vi "fit -- freq vs T - V3.vi"(0 "time points":dbl[](array[numeric]), 1 "varshni win (relative)":dbl=1.25, 2 "fit using":T1=enum."varshni", 5 "temperature points":dbl[](array[numeric]), 9 "frequency points":dbl[](array[numeric]), 11 "cursor bracket: freq":T2={"left"=2378.60310421286, "right "=2421.6740576496672, "center"=2421.6740576496672, "window"=2421.6740576496672, "cursors"=[], "relative"=0, "absolute"=0, "fixed vertical offset"=2421.6740576496672, "vertical offset"=2421.6740576496672, "skew"=2421.6740576496672, "default window frac"=2421.6740576496672, "kind"=enum."skewed", "skew.left"=2421.6740576496672, "skew.right"=2421.6740576496672, "Plot ref"=refnum, "wing order"=enum."back"}, 12 "redo for varshni window?":bool) -> (3 "best fit parameters":dbl[](array[numeric])=[1510.033618014085, -0.06734487332989668, -59.94387240978006], 4 "fit function name":string="fit function - varshni3.vi", 13 "fit points before":i32=434, 14 "fit points after":i32=434)   [LabVIEW 2015]
uses:
  D:/github/resonant_ultrasound/maglab ultrasound -- arkady/cursor winow.ctl
  fit function selector control.ctl
  <vilib>/gmath/NumericalOptimization/Nonlinear Curve Fit LM.vi
  <vilib>/gmath/NI_Gmath.lvlib
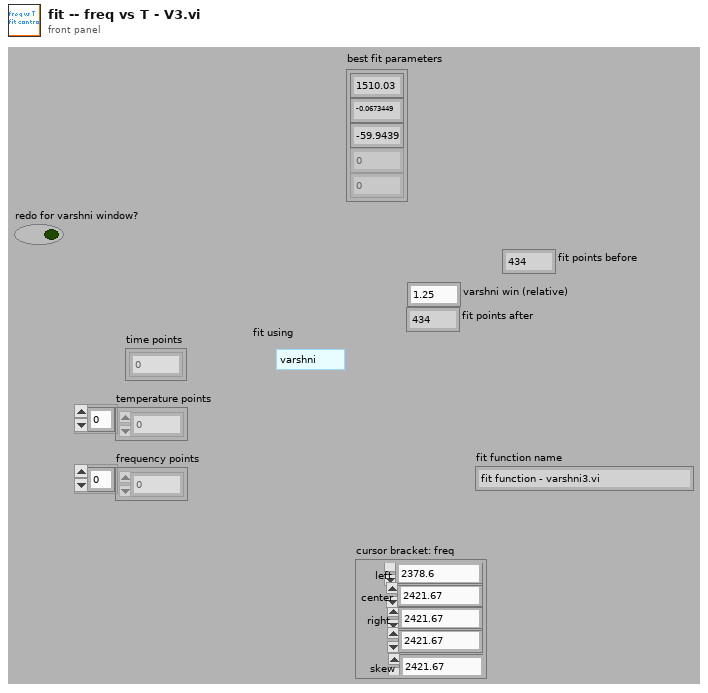
[diagram p1: front panel]
types:
  T1 = typedef "fit function selector control.ctl" = enum16{"linear", "varshni", "varshni5", "LogMinusT", "hyperbola", "einstein", "sine", "sine2theta", "cos2theta"}
  T2 = typedef "cursor winow.ctl" = cluster{"left":dbl, "right ":dbl, "center":dbl, "window":dbl, "cursors":i32[], "relative":i32, "absolute":i32, "fixed vertical offset":dbl, "vertical offset":dbl, "skew":dbl, "default window frac":dbl, "kind":enum16{"symmetric", "skewed", "fancy"}, "skew.left":dbl, "skew.right":dbl, "Plot ref":refnum<vi>, "wing order":enum16{"forw", "back"}}
  T3 = cluster{"model":string, "Parameters":string[], "x":string}
  T4 = typedef "NI_Gmath.lvlib/LM model function reference.ctl" = refnum<vi>
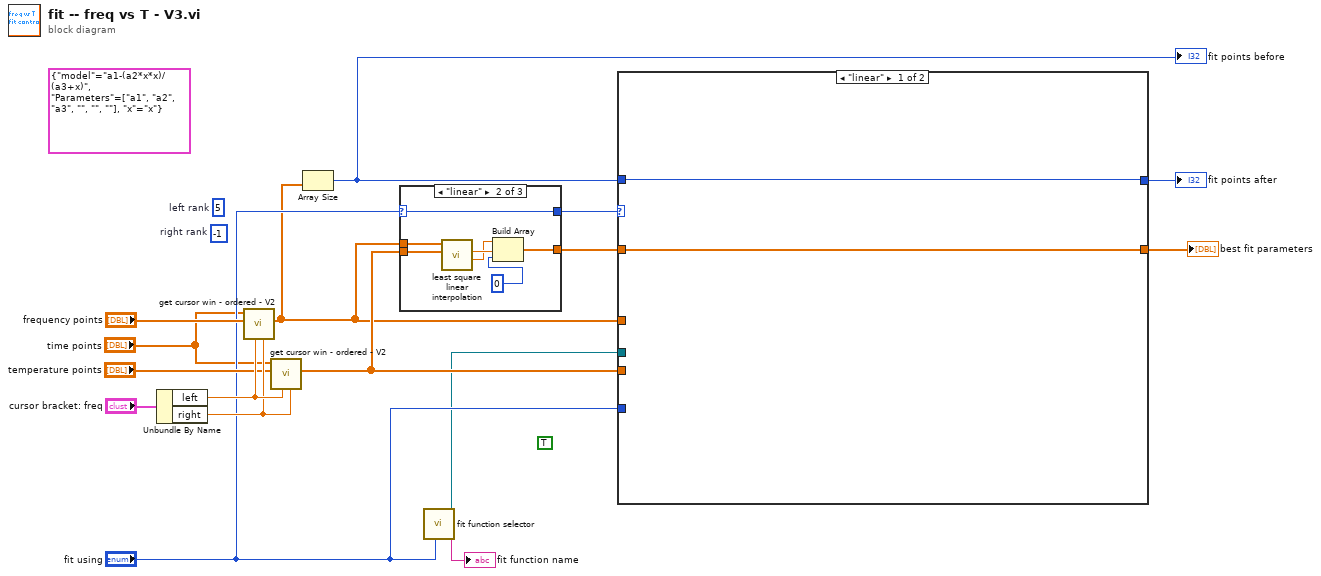
[diagram p0: block diagram]
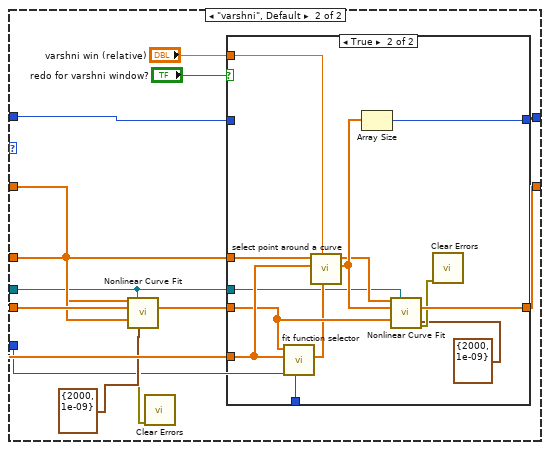
[diagram p2: hidden frame]
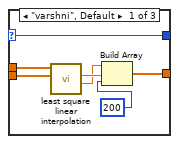
[diagram p4: hidden frame]
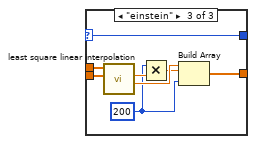
[diagram p5: hidden frame]
diagram:
  (unwired) T3 {"model"="a1-(a2*x*x)/(a3+x)", "Parameters"=["a1", "a2", "a3", "", "", ""], "x"="x"} ("model description")
  (unwired) TRUE
  (unwired) -1  # right rank
  (unwired) 5  # left rank
  n1 = Unbundle By Name("cursor bracket: freq") -> ("left"=w14:dbl, "right"=w13:dbl)
  n2 = call "get cursor win - ordered - V2.vi"("right"=w13, "left"=w14, "freq"="frequency points", "time points"="time points") -> ("freq out"=w4:dbl[])  [unwired: 6 in, 1 out]
  n3 = call "get cursor win - ordered - V2.vi"("right"=w13, "left"=w14, "freq"="temperature points", "time points"="time points") -> ("freq out"=w9:dbl[])  [unwired: 6 in, 1 out]
  n4 = Array Size(array=w4) -> (size(s)=w2:i32)
  "fit points before" <- w2
  n5 = case shown="\"linear\"" "fit using" {
    selector: "fit using" -> [w17 w24 w31]
    tunnel: w9 -> [w23 w30 w38]
    tunnel: w4 -> [w22 w29 w37]
    tunnel: [w20 w27 w36] -> w8
    tunnel: [w17 w24 w31] -> w1
    frame "varshni", Default {
      n6 = call "least square linear interpolation.vi"("X"=w23, "Y"=w22) -> ("intercept"=w18:dbl, "slope"=w19:dbl)  [unwired: 8 in]
      n7 = Build Array(w18, w19, 200) -> (w20:dbl[])
    }
    frame "linear" {
      n8 = call "least square linear interpolation.vi"("X"=w30, "Y"=w29) -> ("intercept"=w25:dbl, "slope"=w26:dbl)  [unwired: 8 in]
      n9 = Build Array(w25, w26, 0) -> (w27:dbl[])
    }
    frame "einstein" {
      w33 = 200
      n10 = call "least square linear interpolation.vi"("X"=w38, "Y"=w37) -> ("intercept"=w35:dbl, "slope"=w34:dbl)  [unwired: 8 in]
      n11 = Multiply(x=w33, y=w34) -> (x*y=w32:dbl)
      n12 = Build Array(w35, w32, w33) -> (w36:dbl[])
    }
  }
  n13 = call "fit function selector.vi"("fit using"="fit using") -> ("fit function name"=→"fit function name":string, "vi reference"=w3:T4)  [unwired: 8 in, 1 out]
  n14 = case shown="\"linear\"" w1 {
    tunnel: [w40 w52] -> w12
    tunnel: [w39 w51] -> w11
    tunnel: w9 -> [_ w50]
    tunnel: w8 -> [w40 w46]
    tunnel: "fit using" -> [_ w45]
    tunnel: w4 -> [_ w44]
    tunnel: w3 -> [_ w43]
    tunnel: w2 -> [w39 w41]
    frame "linear" {
    }
    frame "varshni", Default {
      n15 = call-poly <vilib>:"Nonlinear Curve Fit.vi"("Y"=w44, "f(x,a)"=w43, "X"=w50, "initial parameters"=w46, "termination"=cluster{"max iteration":i32, "tolerance":dbl} {"max iteration"=2000, "tolerance"=1e-09}) -> ("best fit parameters"=w47:dbl[], "error out"=w48:errorcluster)  [unwired: 5 in, 4 out]
      n16 = call <vilib>:"Clear Errors.vi"("error in (no error)"=w48) -> ()  [unwired: 5 in, 2 out]
      n17 = case shown="True" "redo for varshni window?" {
        tunnel: "varshni win (relative)" -> [_ w68]
        tunnel: [w55 w67] -> w52
        tunnel: [w54 w66] -> w51
        tunnel: w50 -> [_ w65]
        tunnel: w47 -> [w55 w62]
        tunnel: w45 -> [_ w58]
        tunnel: w44 -> [_ w57]
        tunnel: w43 -> [_ w56]
        tunnel: w41 -> [w54 _]
        frame False {
        }
        frame True {
          n18 = call "fit function selector.vi"("fit using"=w58, "temperature"=w65, "best fit parameters"=w62) -> ("freq out"=w59:dbl[])  [unwired: 6 in, 2 out]
          n19 = call "select point around a curve.vi"("freq  ref curve"=w59, "window"=w68, "temperature"=w65, "freq"=w57) -> ("temperature  out"=w61:dbl[], "freq out"=w60:dbl[])  [unwired: 6 in]
          n20 = Array Size(array=w61) -> (size(s)=w66:i32)
          n21 = call-poly <vilib>:"Nonlinear Curve Fit.vi"("Y"=w60, "f(x,a)"=w56, "X"=w61, "initial parameters"=w62, "termination"=cluster{"max iteration":i32, "tolerance":dbl} {"max iteration"=2000, "tolerance"=1e-09}) -> ("best fit parameters"=w67:dbl[], "error out"=w64:errorcluster)  [unwired: 5 in, 4 out]
          n22 = call <vilib>:"Clear Errors.vi"("error in (no error)"=w64) -> ()  [unwired: 5 in, 2 out]
        }
      }
    }
  }
  "best fit parameters" <- w12
  "fit points after" <- w11
